vi "parse_uint32.vi"   [LabVIEW 2018]
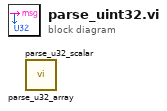
[diagram p0: block diagram]
diagram:
  n1 = call <userlib>:"parse_u32_array.vi"() -> ()  [unwired: 5 in, 3 out]
  n2 = call <userlib>:"parse_u32_scalar.vi"() -> ()  [unwired: 5 in, 3 out]
